vi "_Main.vi"() -> ()   [LabVIEW 2017, in "Overlords.lvlib"]
uses:
  Overlords.lvlib
  Cluster_CMD to SM Data.ctl
  Hopper/ENUM_Firing_State.ctl
  Hopper/Hopper System.lvlib
  <vilib>/Rock Robotics/WPI/DriverStation/WPI_DriverStationMatch Info.ctl
  ENUM_Overloard State.ctl
  Global_CMD Data.vi
  Global_SM_Data Out.vi
  Globals/Global_STOP.vi
  ENUM _Overloard Shooter States.ctl
  ENUM_Overloard Gear States.ctl
  ENUM_Overloard Climb States.ctl
panel:
  out "Overlord Climber State":T1
  out "Overlord Gear State":T2
  out "Overloard Shooter States":T3
  out "Wanted State":T4
  out "Current Overlord State":T4
  out "Task Complete":bool
  in  "Low Shot - Rapid Fire Button":bool
  in  "Low Shot - Shotgun Button":bool
  in  "High Shot - Rapid Fire Button":bool
  in  "High Shot - Shotgun Button":bool
  in  "Gear Button":bool
  in  "Climb Button":bool
  in  "Match Info":T5={"Autonomous Elapsed Seconds"=0.0, "TeleOp Elapsed Seconds"=0.0, "Disabled Elapsed Seconds"=0.0, "Visited Autonomous"=FALSE, "Visited TeleOp"=FALSE, "Visited Disabled"=FALSE, "Autonomous Settings"={"Autonomous Style"=enum."Independent", "VI Refnum"=refnum}}
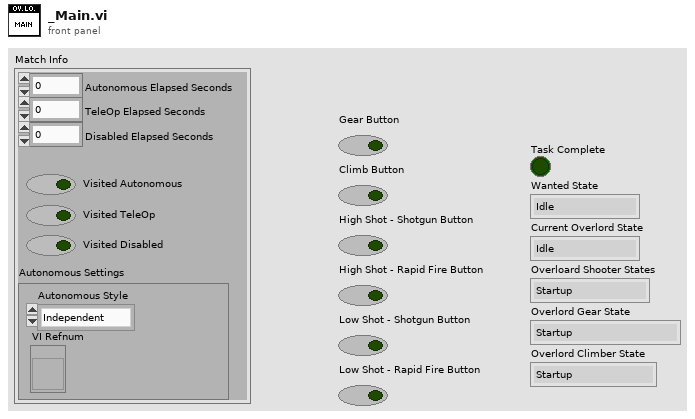
[diagram p1: front panel]
types:
  T1 = typedef "Overlords.lvlib/ENUM_Overloard Climb States.ctl" = enum16{"Startup", "Idle", "Check Time", "Check Statis", "Complete"}
  T2 = typedef "Overlords.lvlib/ENUM_Overloard Gear States.ctl" = enum16{"Startup", "Idle", "Detect Target", "Verticle Track (Sonar)", "Encoder Setup", "Verticle Track (Encoder)", "Gear Present", "Gear Present Counter", "Verticle Backword Track", "Complete"}
  T3 = typedef "Overlords.lvlib/ENUM _Overloard Shooter States.ctl" = enum16{"Startup", "Idle", "Locate Target", "Wait To Be in Position", "Shooting", "Complete"}
  T4 = typedef "Overlords.lvlib/ENUM_Overloard State.ctl" = enum16{"Idle", "High Shot", "Low Shot", "Place Gear", "Climb"}
  T5 = typedef "WPI_DriverStationMatch Info.ctl" = cluster{"Autonomous Elapsed Seconds":dbl, "TeleOp Elapsed Seconds":dbl, "Disabled Elapsed Seconds":dbl, "Visited Autonomous":bool, "Visited TeleOp":bool, "Visited Disabled":bool, "Autonomous Settings":cluster{"Autonomous Style":enum16{"Iterative", "Independent"}, "VI Refnum":refnum<vi>}}
  T6 = typedef "Overlords.lvlib/Cluster_CMD to SM Data.ctl" = cluster{"Overloard State":T4, "Match Info":T5, "Firing State":T7, "Gear wait till pullback (seconds)":dbl}
  T7 = typedef "Hopper System.lvlib/ENUM_Firing_State.ctl" = enum16{"No Fireing", "Rapid Fire", "Shotgun Fireing"}
  T8 = typedef "Overlords.lvlib/Cluster_SM Status.ctl" = cluster{"Task Complete":bool, "Current Overlord State":T4, "Wanted State":T4, "Overloard Shooter States":T3, "Overlord Gear State":T2, "Overlord Climber State":T1}
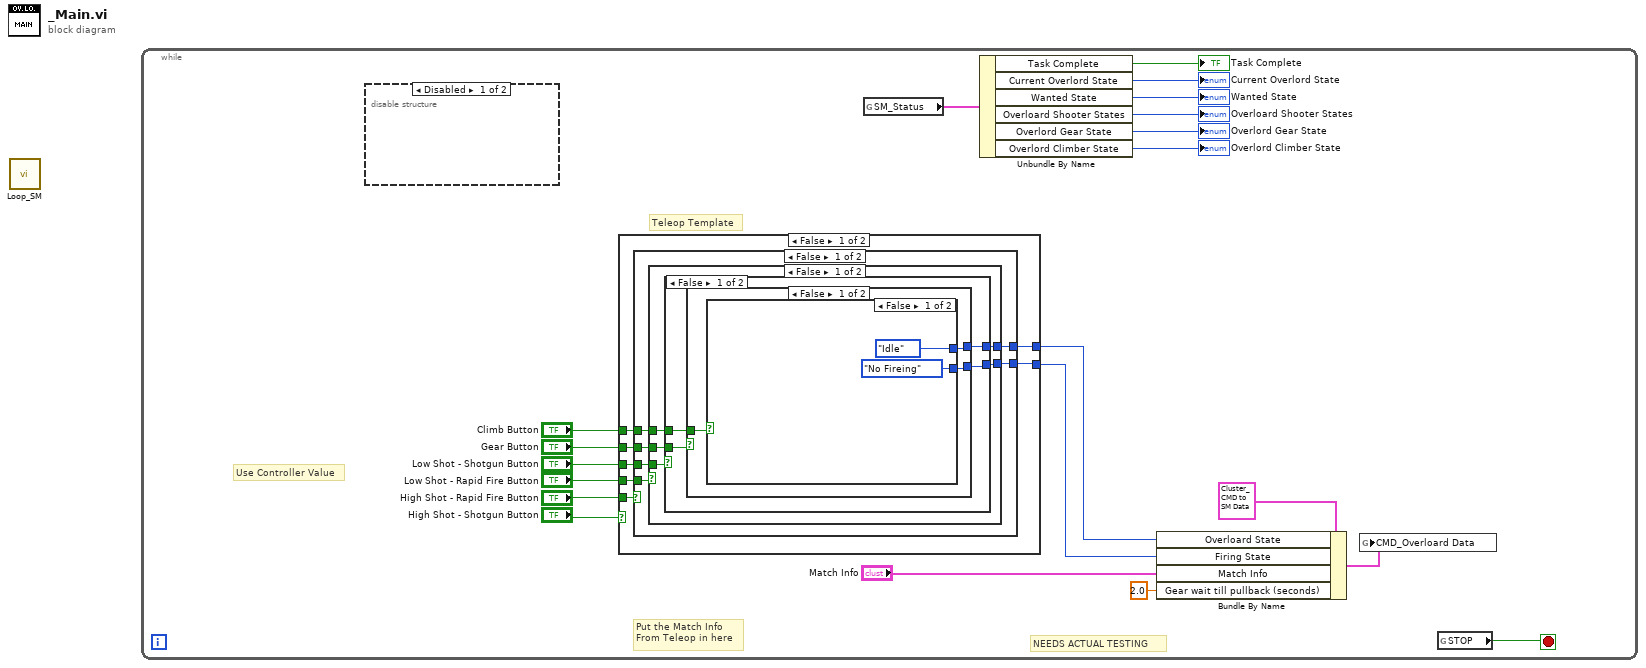
[diagram p0: block diagram]
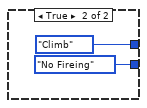
[diagram p2: hidden frame]
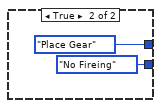
[diagram p3: hidden frame]
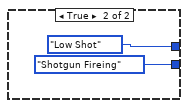
[diagram p4: hidden frame]
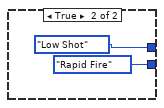
[diagram p5: hidden frame]
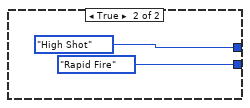
[diagram p6: hidden frame]
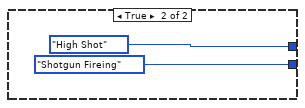
[diagram p7: hidden frame]
diagram:
  n1 = call "Loop_SM.vi"() -> ()  [unwired: 12 in]
  n2 = while {
    stop <- w1 stop-if-true
    # "Teleop Template"
    # "Use Controller Value"
    # "NEEDS ACTUAL TESTING"
    # "Put the Match Info\nFrom Teleop in here"
    n3 = disable-structure shown="Disabled" {
      frame Disabled {
      }
      frame Enabled {
      }
    }
    n4 = case shown="False" "High Shot - Shotgun Button" {
      tunnel: [w26 ENUM_Overloard_State."High Shot" ("Overloard State")] -> w11
      tunnel: [w25 ENUM_Firing_State."Shotgun Fireing" ("Firing State")] -> w10
      tunnel: "High Shot - Rapid Fire Button" -> [w27 _]
      tunnel: "Low Shot - Rapid Fire Button" -> [w24 _]
      tunnel: "Low Shot - Shotgun Button" -> [w23 _]
      tunnel: "Gear Button" -> [w22 _]
      tunnel: "Climb Button" -> [w21 _]
      frame False {
        n5 = case shown="False" w27 {
          tunnel: [w32 ENUM_Overloard_State."High Shot" ("Overloard State")] -> w26
          tunnel: [w31 ENUM_Firing_State."Rapid Fire" ("Firing State")] -> w25
          tunnel: w24 -> [w33 _]
          tunnel: w23 -> [w30 _]
          tunnel: w22 -> [w29 _]
          tunnel: w21 -> [w28 _]
          frame False {
            n6 = case shown="False" w33 {
              tunnel: [w37 ENUM_Overloard_State."Low Shot" ("Overloard State")] -> w32
              tunnel: [w36 ENUM_Firing_State."Rapid Fire" ("Firing State")] -> w31
              tunnel: w30 -> [w38 _]
              tunnel: w29 -> [w35 _]
              tunnel: w28 -> [w34 _]
              frame False {
                n7 = case shown="False" w38 {
                  tunnel: [w41 ENUM_Overloard_State."Low Shot" ("Overloard State")] -> w37
                  tunnel: [w40 ENUM_Firing_State."Shotgun Fireing" ("Firing State")] -> w36
                  tunnel: w35 -> [w42 _]
                  tunnel: w34 -> [w39 _]
                  frame False {
                    n8 = case shown="False" w42 {
                      tunnel: [w44 ENUM_Overloard_State."Place Gear" ("Overloard State")] -> w41
                      tunnel: [w43 ENUM_Firing_State."No Fireing" ("Firing State")] -> w40
                      tunnel: w39 -> [w45 _]
                      frame False {
                        n9 = case shown="False" w45 {
                          tunnel: [ENUM_Overloard_State."Idle" ("Overloard State") ENUM_Overloard_State."Climb" ("Overloard State")] -> w44
                          tunnel: [ENUM_Firing_State."No Fireing" ("Firing State") ENUM_Firing_State."No Fireing" ("Firing State")] -> w43
                          frame False {
                          }
                          frame True {
                          }
                        }
                      }
                      frame True {
                      }
                    }
                  }
                  frame True {
                  }
                }
              }
              frame True {
              }
            }
          }
          frame True {
          }
        }
      }
      frame True {
      }
    }
    n10 = global read "Global_SM_Data Out.vi" "SM_Status"() -> (w8:T8)
    n11 = Unbundle By Name(w8) -> ("Task Complete"=→"Task Complete":bool, "Current Overlord State"=→"Current Overlord State":T4, "Wanted State"=→"Wanted State":T4, "Overloard Shooter States"=→"Overloard Shooter States":T3, "Overlord Gear State"=→"Overlord Gear State":T2, "Overlord Climber State"=→"Overlord Climber State":T1)
    n12 = Bundle By Name(cluster=T6 {"Overloard State"=enum."Idle", "Match Info"={"Autonomous Elapsed Seconds"=0.0, "TeleOp Elapsed Seconds"=0.0, "Disabled Elapsed Seconds"=0.0, "Visited Autonomous"=FALSE, "Visited TeleOp"=FALSE, "Visited Disabled"=FALSE, "Autonomous Settings"={"Autonomous Style"=enum."Independent", "VI Refnum"=refnum}}, "Firing State"=enum."No Fireing", "Gear wait till pullback (seconds)"=0.0} ("CMD_Overloard Data"), "Overloard State"=w11, "Firing State"=w10, "Match Info"="Match Info", "Gear wait till pullback (seconds)"=2.0) -> (w20:T6)
    n13 = global write "Global_CMD Data.vi" "CMD_Overloard Data"(w20) -> ()
    n14 = global read "Global_STOP.vi" "STOP"() -> (w1:bool)
  }
